vi "Dispatch Shutdown.vi"(8 "error in (no error)":errorcluster, 11 "Dispatcher in":refnum<class "Dispatcher Thread.lvclass">) -> (0 "error out":errorcluster, 3 "Dispatcher out":refnum<class "Dispatcher Thread.lvclass">)   [LabVIEW 2017, in "DSF Core.lvlib" / "Dispatcher Thread.lvclass"]
uses:
  Dispatcher Thread.lvclass
  C:/Git/DSF/Data Sharing Framework Core/Classes/Thread/Thread.lvclass
  Dispatcher Thread.lvclass/Dispatcher Thread.ctl
  Thread Pool/Plugin Interface Pool.lvclass/Plugin Interface Pool.ctl
  Interfaces/Dispatcher/Response Data.ctl
  Interfaces/Dispatcher/Response.ctl
  Interfaces/Dispatcher/Parameters.ctl
  Interfaces/Dispatcher/Write Dispatcher Response.vi
  Thread Pool/Plugin Interface Pool.lvclass
  Interfaces/Plugin/Plugin Interface.lvclass
  Thread/Thread.lvclass
  Interfaces/Dispatcher/Dispatcher Interface.lvclass
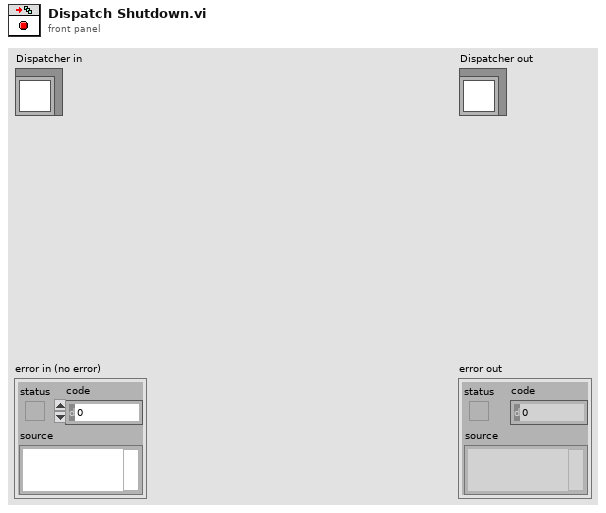
[diagram p1: front panel]
types:
  T1 = typedef "DSF Core.lvlib/Dispatcher Thread.lvclass/Plugin Settings.ctl" = cluster{"Transfer Group threads":i32[], "Plugin Thread Pool":refnum<class "Plugin Interface Pool.lvclass">}
  T2 = typedef "DSF Core.lvlib/Dispatcher Interface.lvclass/Response Data.ctl" = cluster{"Response":T3, "Parameters":T4}
  T3 = typedef "DSF Core.lvlib/Dispatcher Interface.lvclass/Response.ctl" = enum8{"General Ack", "Error", "Shutting Down"}
  T4 = typedef "DSF Core.lvlib/Dispatcher Interface.lvclass/Parameters.ctl" = cluster{"arg1":u64, "arg2":u64}
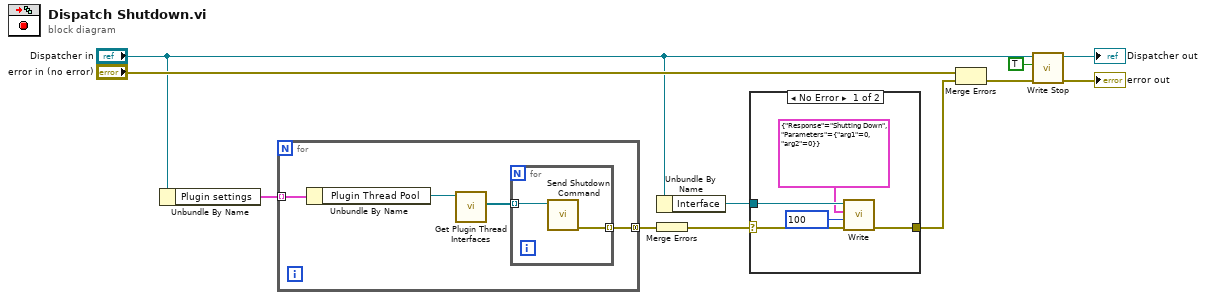
[diagram p0: block diagram]
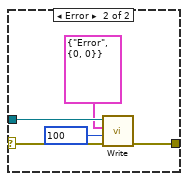
[diagram p2: hidden frame]
diagram:
  n1 = Unbundle By Name("Dispatcher in") -> ("Plugin settings"=w11:T1[])
  n2 = for {
    tunnel: w11 -> [w15] mode=indexing
    tunnel: [w12] -> w10 mode=concatenating
    n3 = Unbundle By Name(w15) -> ("Plugin Thread Pool"=w14:refnum<class "Plugin Interface Pool.lvclass">)
    n4 = call "Get Plugin Thread Interfaces.vi"("Plugin Interface Pool in"=w14) -> ("Plugin Thread Interfaces"=w13:refnum<class "Plugin Interface.lvclass">[])  [unwired: 9 in, 1 out]
    n5 = for {
      tunnel: w13 -> [w17] mode=indexing
      tunnel: [w16] -> w12 mode=indexing
      n6 = call "Send Shutdown Command.vi"("Plugin Interface in"=w17) -> ("error out"=w16:errorcluster)  [unwired: 9 in, 1 out]
    }
  }
  n7 = Unbundle By Name("Dispatcher in") -> ("Interface"=w3:refnum<class "Dispatcher Interface.lvclass">)
  n8 = Merge Errors(w10) -> (w6:errorcluster)
  n9 = case shown="No Error" w6 {
    selector: w6 -> [w20 w25]
    tunnel: [w21 w26] -> w5
    tunnel: w3 -> [w19 w24]
    frame No Error {
      n10 = call-poly "Write.vi"("error in (no error)"=w20, "timeout in ms (0)"=100, "response"=T2 {"Response"=enum."Shutting Down", "Parameters"={"arg1"=0, "arg2"=0}}, "Dispatcher Interface in"=w19) -> ("error out"=w21:errorcluster)  [unwired: 6 in, 1 out]
    }
    frame Error {
      n11 = call-poly "Write.vi"("error in (no error)"=w25, "timeout in ms (0)"=100, "response"=T2 {"Response"=enum."Error", "Parameters"={"arg1"=0, "arg2"=0}}, "Dispatcher Interface in"=w24) -> ("error out"=w26:errorcluster)  [unwired: 6 in, 1 out]
    }
  }
  n12 = Merge Errors("error in (no error)", w5) -> (w4:errorcluster)
  n13 = call "Write Stop.vi"("error in (no error)"=w4, "stop"=TRUE, "Thread in"="Dispatcher in") -> ("error out"=→"error out":errorcluster, "Thread out"=→"Dispatcher out":refnum<class "Dispatcher Thread.lvclass">)  [unwired: 7 in]
